vi "Raster 1.vi"() -> ()   [LabVIEW 2022 SP3, in "Benchmark.lvlib"]
uses:
  Benchmark.lvlib
  <vilib>/Analysis/NI_AALBase.lvlib
panel:
  out "Std Dev":dbl format="%.1p"
  out "Mean":dbl format="%.1p"
  out "Histogram Graph":T1(graph)
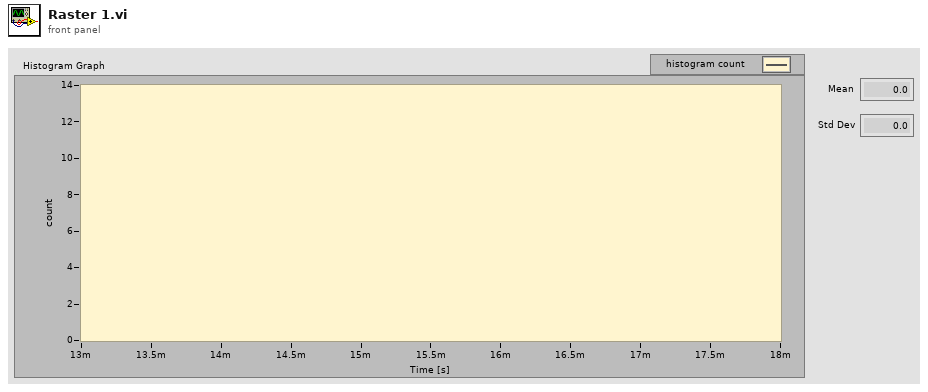
[diagram p1: front panel]
types:
  T1 = cluster{"X Values":dbl[], "Histogram: h(x)":i32[]}
  T2 = typedef "Core Data.ctl" = cluster{"Screen Dimensions":T3, "Camera":T4, "Transform":T5, "Line Colour":u32, "Fill Colour":u32, "Draw Lines":bool, "Projection Matrix":sgl[][], "Update Screen":bool, "Frame Buffer":refnum<data-value>, "Objects":T7[], "Camera Up":sgl, "Camera Left":sgl, "Camera Rotation":sgl, "Camera Forward":sgl, "Draw Triangles":bool, "Frame Buffer 2":refnum<data-value>, "Framebuffer":bool, "Pixel Data 1":u32[][]}
  T3 = typedef "Raster.lvlib/Screen Dimensions.ctl" = cluster{"Width":u32, "Height":u32}
  T4 = typedef "3D.lvlib/Camera.ctl" = cluster{"Field Of View":sgl, "Near Plane":sgl, "Far Plane":sgl}
  T5 = typedef "3D.lvlib/Transform.ctl" = cluster{"Position":T6, "Rotation":T6, "Scale":T6}
  T6 = typedef "3D.lvlib/Vector 3D.ctl" = cluster{"x":sgl, "y":sgl, "z":sgl}
  T7 = typedef "3D.lvlib/Mesh.ctl" = cluster{"Triangles":T8[]}
  T8 = typedef "3D.lvlib/Triangle 3D.ctl" = cluster{"Point 1":T6, "Point 2":T6, "Point 3":T6, "Fill Colour":u32}
  T9 = typedef "3D.lvlib/Triangle 2D.ctl" = cluster{"Point 1":T10, "Point 2":T10, "Point 3":T10, "Fill Colour":u32}
  T10 = typedef "3D.lvlib/Point 2D.ctl" = cluster{"x":sgl, "y":sgl}
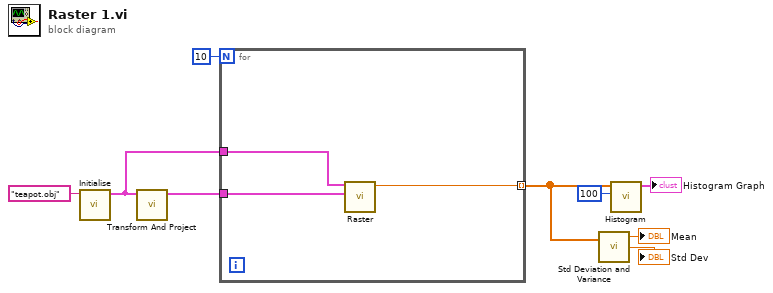
[diagram p0: block diagram]
diagram:
  n1 = call "Initialise.vi"("name or relative path"="teapot.obj") -> ("Core Data"=w1:T2)  [unwired: 9 in, 1 out]
  n2 = call "Transform And Project.vi"("Core Data"=w1) -> ("Triangles Sorted"=w2:T9[])  [unwired: 9 in, 1 out]
  n3 = for {
    N: 10 -> [_]
    tunnel: w2 -> [w11]
    tunnel: [w10] -> w5 mode=indexing
    tunnel: w1 -> [w12]
    n4 = call "Raster.vi"("Triangles Sorted"=w11, "Core Data in"=w12) -> ("Delta Time [s]"=w10:dbl)  [unwired: 8 in, 1 out]
  }
  n5 = call <vilib>:"Std Deviation and Variance.vi"("X"=w5) -> ("mean"=→"Mean":dbl, "standard deviation"=→"Std Dev":dbl)  [unwired: 1 in, 1 out]
  n6 = call <vilib>:"Histogram.vi"("intervals"=100, "X"=w5) -> ("Histogram Graph"=→"Histogram Graph":T1)  [unwired: 6 in, 3 out]
